vi "MGI Top Level VI Reference.vi"() -> (0 "Top Level VI Reference":refnum<vi>)   [LabVIEW 2016]
doc: "Returns a reference to the top level VI.\n\nAuthored by Robert C. Mortensen\nsupport@mooregoodideas.com\nwww.mooregoodideas.com\n\nCopyright (c) 2010, Moore Good Ideas, Inc.\n\nAll rights reserved.\n\nRedistribution and use in source and binary forms, with or without modification, are permitted provided that the following conditions are met:\n\n * Redistributions of source code must retain the above copyright notice, this list of conditions and the following disclaimer.\n * Redistributions in binary form must reproduce the above copyright notice, this list of conditions and the following disclaimer in the documentation and/or other materials provided with the distribution.\n * Neither the name of Moore Good Ideas, Inc. nor the names of its contributors may be used to endorse or promote products derived from this software without specific prior written permission.\n\nTHIS SOFTWARE IS PROVIDED BY THE COPYRIGHT HOLDERS AND CONTRIBUTORS \"AS IS\" AND ANY EXPRESS OR IMPLIED WARRANTIES, INCLUDING, BUT NOT LIMITED TO, THE IMPLIED WARRANTIES OF MERCHANTABILITY AND FITNESS FOR A PARTICULAR PURPOSE ARE DISCLAIMED. IN NO EVENT SHALL THE COPYRIGHT OWNER OR CONTRIBUTORS BE LIABLE FOR ANY DIRECT, INDIRECT, INCIDENTAL, SPECIAL, EXEMPLARY, OR CONSEQUENTIAL DAMAGES (INCLUDING, BUT NOT LIMITED TO, PROCUREMENT OF SUBSTITUTE GOODS OR SERVICES; LOSS OF USE, DATA, OR PROFITS; OR BUSINESS INTERRUPTION) HOWEVER CAUSED AND ON ANY THEORY OF LIABILITY, WHETHER IN CONTRACT, STRICT LIABILITY, OR TORT (INCLUDING NEGLIGENCE OR OTHERWISE) ARISING IN ANY WAY OUT OF THE USE OF THIS SOFTWARE, EVEN IF ADVISED OF THE POSSIBILITY OF SUCH DAMAGE."
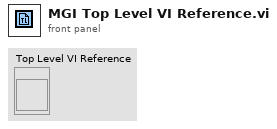
[diagram p1: front panel]
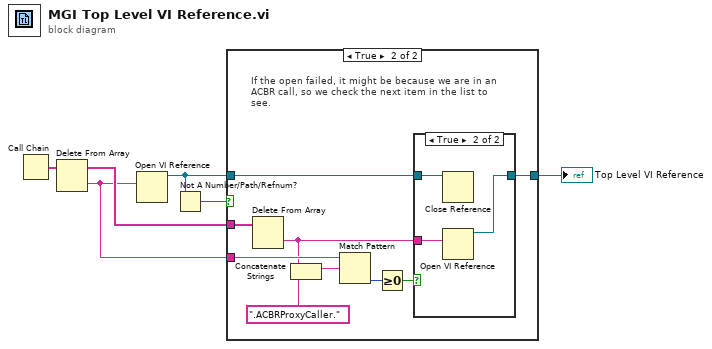
[diagram p0: block diagram]
diagram:
  n1 = Call Chain() -> (call chain=w6:string[])
  n2 = Delete From Array(array=w6) -> (deleted portion=w1:string, array with subset deleted=w4:string[])  [unwired: 2 in]
  n3 = Open VI Reference(vi path=w1) -> (vi reference=w3:refnum<vi>)  [unwired: 5 in, 1 out]
  n4 = Not A Number/Path/Refnum?(number/path/refnum=w3) -> (NaN/Path/Refnum?=w5:bool)
  n5 = case shown="True" w5 {
    tunnel: w4 -> [_ w16]
    tunnel: w3 -> [w7 w15]
    tunnel: [w7 w14] -> w2
    tunnel: w1 -> [_ w11]
    frame False {
    }
    frame True {
      # "If the open failed, it might be because we are in an ACBR call, so we check the next item in the list to see."
      n6 = Delete From Array(array=w16) -> (deleted portion=w8:string)  [unwired: 2 in, 1 out]
      n7 = Concatenate Strings(w8, ".ACBRProxyCaller.") -> (w13:string)
      n8 = Match Pattern(string=w11, regular expression=w13) -> (offset past match=w10:i32)  [unwired: 1 in, 3 out]
      n9 = Greater Or Equal To 0?(x=w10) -> (x >= 0?=w9:bool)
      n10 = case shown="True" w9 {
        tunnel: w15 -> [w17 w20]
        tunnel: [w17 w19] -> w14
        tunnel: w8 -> [_ w18]
        frame False {
        }
        frame True {
          n11 = Close Reference(reference=w20) -> ()  [unwired: 1 in, 1 out]
          n12 = Open VI Reference(vi path=w18) -> (vi reference=w19:refnum<vi>)  [unwired: 5 in, 1 out]
        }
      }
    }
  }
  "Top Level VI Reference" <- w2
